vi "Write Variant.vi"(8 "error in (no error)":errorcluster, 9 "Variant":variant, 10 "Tag":string, 11 "Omni_Bus in":refnum<class "Omni_Bus.lvclass">) -> (0 "error out":errorcluster, 3 "Omni_Bus out":refnum<class "Omni_Bus.lvclass">)   [LabVIEW 2021, in "Omni_Bus.lvclass"]
uses:
  Omni_Bus.lvclass
  Omni_Bus.lvclass/Omni_Bus.ctl
  <vilib>/TSA/Abstract Data Classes/Abs_Types/Variant/Abs_Variant.lvclass
  C:/Program Files (x86)/National Instruments/LabVIEW 2021/vi.lib/TSA/Abstract Data Classes/Abs_Types/Value/Abs_Value.lvclass
  C:/Program Files (x86)/National Instruments/LabVIEW 2021/vi.lib/TSA/Abstract Data Classes/Abs_Types/Type/Abs_Type.lvclass
  C:/Program Files (x86)/National Instruments/LabVIEW 2021/vi.lib/TSA/Abstract Data Classes/Abs_Types/Variant/Abs_Variant.lvclass
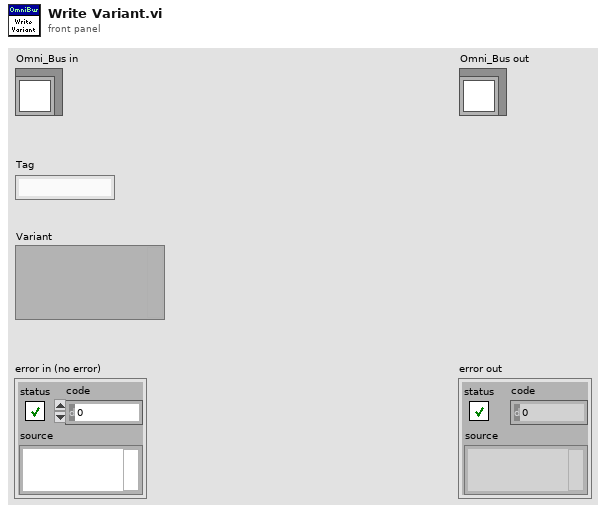
[diagram p1: front panel]
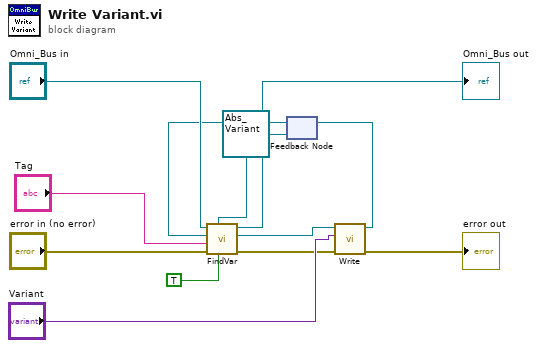
[diagram p0: block diagram]
diagram:
  w1 = refnum<class "Abs_Variant.lvclass"> refnum ("Abs_Variant out")
  n1 = feedback #1(w1) -> (w3:refnum<class "Abs_Variant.lvclass">)
  n2 = call "FindVar.vi"("Write?"=TRUE, "Abs_Type"=w1, "error in (no error)"="error in (no error)", "Tag"="Tag", "Abs_Type Default"=w3, "Var Bus in"="Omni_Bus in") -> ("error out"=w6:errorcluster, "Abs_Type Found"=w4:refnum<class "Abs_Variant.lvclass">, "Var Bus out"=→"Omni_Bus out":refnum<class "Omni_Bus.lvclass">)  [unwired: 2 in, 1 out]
  n3 = call-dynamic "Write.vi"("error in (no error)"=w6, "Variant"="Variant", "Abs_Variant in"=w4) -> ("error out"=→"error out":errorcluster, "Abs_Variant out"=w5:refnum<class "Abs_Variant.lvclass">)  [unwired: 7 in]
  n4 = feedback-in #1(w5) -> ()
